vi "Configure Session.vi"(8 "error in (no error)":errorcluster, 11 "RandomNumberLogger in":refnum<class "RandomNumberLogger.lvclass">) -> (0 "error out":errorcluster, 3 "RandomNumberLogger out":refnum<class "RandomNumberLogger.lvclass">)   [LabVIEW 2020, in "RandomNumberLogger.lvlib" / "RandomNumberLogger.lvclass"]
doc: "<b>Configure Session</b>\nCalled once per session, and is always called after the plugin loads its configuration\n\nFor the ADAS use case, we typically only have a single session of a plugin during a run. In the future we may add the ability to support multiple sessions.\n\nIn this VI, take the configuration parameters and call the appropriate initialization functions to open and store any references needed during the run. For example, call Open/Create/Replace File on the path stored in configuration and store the file reference as part of the class private data for the plugin class.\n\nIf your plugin needs information from the configuration to decide what timing parameters to use (for example, to configure the period of a Periodic timing), set those here instead of in the Initialize function."
uses:
  RandomNumberLogger.lvclass
  RandomNumberLogger.lvclass/RandomNumberLogger.ctl
  <vilib>/ADAS Record/Utilities/ADAS Utilities.lvlib
  C:/Program Files/National Instruments/LabVIEW 2020/vi.lib/FlexLogger/SDK/PluginSDK.lvlibp/PEFClasses/SDK/Processing Element/Processing Element.lvclass
  C:/Projects/GitHub/data-record-ad/IO Plugins/Tutorial Solutions/RandomNumberLogger/PE/RandomNumberLogger.lvclass
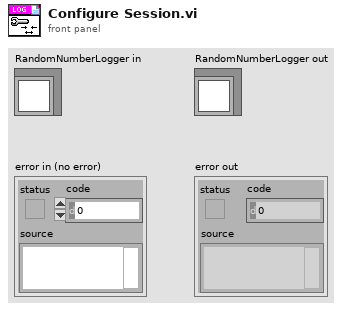
[diagram p1: front panel]
types:
  T1 = typedef "RandomNumberLogger.lvlib/RandomNumberLogger.lvclass/Configuration.ctl" = cluster{"Base File Name":string, "File Directory":path, "File Split":enum16{"None", "Time", "Size"}, "Split Time/Size (sec/MB)":dbl}
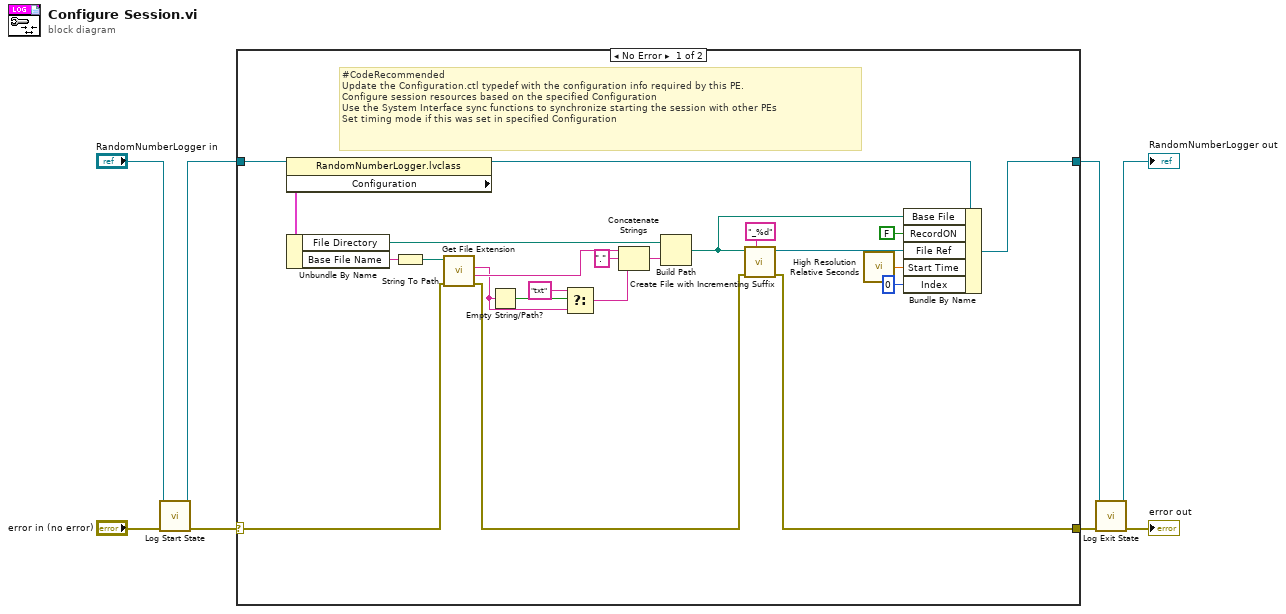
[diagram p0: block diagram]
diagram:
  n1 = call <vilib>:"Log Start State.vi"("error in (no error)"="error in (no error)", "PluginSDK.lvlibp:Processing Element.lvclass"="RandomNumberLogger in") -> ("error out"=w7:errorcluster, "PluginSDK.lvlibp:Processing Element.lvclass"=w5:refnum<class "RandomNumberLogger.lvclass">)  [unwired: 8 in]
  n2 = case shown="No Error" w7 {
    selector: w7 -> [w19 w32]
    tunnel: w5 -> [w31 w33]
    tunnel: [w12 w33] -> w2
    tunnel: [w17 w32] -> w4
    frame No Error {
      # "#CodeRecommended\nUpdate the Configuration.ctl typedef with the configuration info required by this PE.\nConfigure session resources based on the specified Configuration\nUse the System Interface sync functions to synchronize starting the session with other PEs\nSet timing mode if this was set in specified Configuration"
      n3 = property on="Property Node" class="RandomNumberLogger.lvclass"(reference=w31) -> (reference out=w13:refnum<class "RandomNumberLogger.lvclass">, "Configuration"=w30:T1)  [unwired: 1 in, 1 out]
      n4 = Unbundle By Name(w30) -> ("File Directory"=w27:path, "Base File Name"=w29:string)
      n5 = String To Path(string=w29) -> (path=w28:path)
      n6 = call <vilib>:"Get File Extension.vi"("error in (no error)"=w19, "file"=w28) -> ("error out"=w18:errorcluster, "filename without extension"=w25:string, "lowercase file extension"=w21:string)  [unwired: 5 in, 2 out]
      n7 = Empty String/Path?(string/path=w21) -> (empty?=w23:bool)
      n8 = Select(t="txt" ("string"), s=w23, f=w21) -> (s? t:f=w20:string)
      n9 = Concatenate Strings(w25, "." ("string"), w20) -> (w26:string)
      n10 = Build Path(base path=w27, name or relative path=w26) -> (appended path=w9:path)
      n11 = call <vilib>:"Create File with Incrementing Suffix.vi"("format string (\" (%d)\")"="_%d" ("format string (\" (%d)\")"), "error in (no error)"=w18, "file path"=w9) -> ("error out"=w17:errorcluster, "refnum out"=w15:refnum<file>)  [unwired: 6 in, 1 out]
      n12 = call <vilib>:"High Resolution Relative Seconds.vi"() -> ("relative seconds"=w11:dbl)
      n13 = Bundle By Name(cluster=w13, "Base File"=w9, "RecordON"=FALSE, "File Ref"=w15, "Start Time"=w11, "Index"=u64 0) -> (w12:refnum<class "RandomNumberLogger.lvclass">)
    }
    frame Error {
    }
  }
  n14 = call <vilib>:"Log Exit State.vi"("error in (no error)"=w4, "PluginSDK.lvlibp:Processing Element.lvclass"=w2) -> ("error out"=→"error out":errorcluster, "PluginSDK.lvlibp:Processing Element.lvclass"=→"RandomNumberLogger out":refnum<class "RandomNumberLogger.lvclass">)  [unwired: 8 in]
